vi "inspector_state_queue_manager.vi"(8 "error in":errorcluster, 10 "State array in":cluster{"State Enum":T1, "variant":variant}[](array[cluster]), 11 "Inspector_state_queue in":refnum<queue>) -> (0 "error out":errorcluster, 3 "Inspector_state_queue out":refnum<queue>)   [LabVIEW 2010]
uses:
  typedefs/inspector_state_enum.ctl
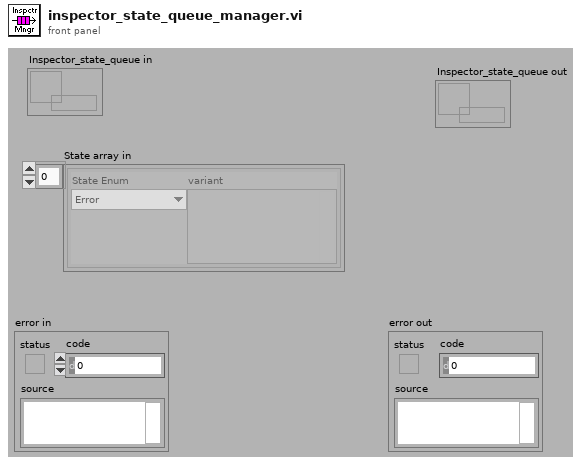
[diagram p1: front panel]
types:
  T1 = typedef "inspector_state_enum.ctl" = enum16{"Init", "Quit", "Error", "ZoomIn", "ZoomOut", "Load", "Change_channel", "Update_graphs"}
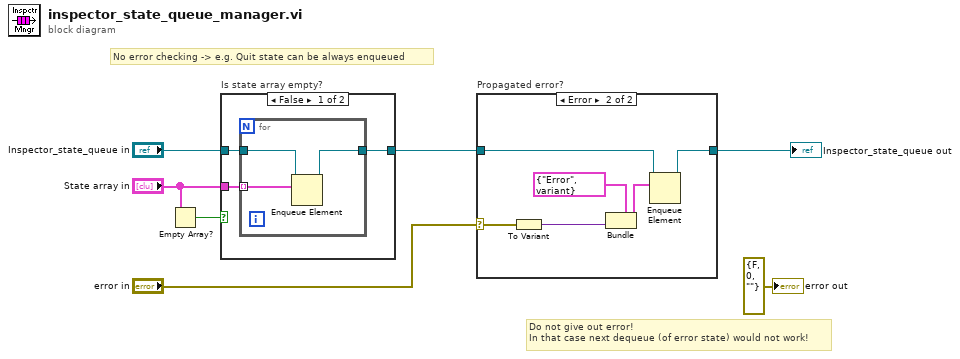
[diagram p0: block diagram]
diagram:
  # "Do not give out error!\nIn that case next dequeue (of error state) would not work!"
  # "No error checking -> e.g. Quit state can be always enqueued"
  n1 = Empty Array?(array="State array in") -> (empty?=w7:bool)
  n2 = case "Is state array empty?" shown="False" w7 {
    tunnel: "Inspector_state_queue in" -> [w10 w14]
    tunnel: [w9 w14] -> w5
    tunnel: "State array in" -> [w8 _]
    frame False {
      n3 = for {
        tunnel: w10 -> [w13]
        tunnel: w8 -> [w12] mode=indexing
        tunnel: [w11] -> w9
        n4 = Enqueue Element(queue=w13, element=w12) -> (queue out=w11:refnum<queue>)  [unwired: 2 in, 2 out]
      }
    }
    frame True {
      # "Empty state array?\nDo not call enqueue\nto avoid errors"
    }
  }
  n5 = case "Propagated error?" shown="Error" "error in" {
    selector: "error in" -> [_ w19]
    tunnel: w5 -> [w15 w21]
    tunnel: [w15 w20] -> w2
    frame No Error {
    }
    frame Error {
      n6 = To Variant(anything=w19) -> (Variant=w17:variant)
      n7 = Bundle(cluster=cluster{"State Enum":T1, "variant":variant} {"State Enum"=enum."Error", "variant"=variant} ("element"), "variant"=w17) -> (w16:cluster{"State Enum":T1, "variant":variant})  [unwired: 1 in]
      n8 = Enqueue Element(queue=w21, element=w16) -> (queue out=w20:refnum<queue>)  [unwired: 2 in, 2 out]
    }
  }
  "Inspector_state_queue out" <- w2
  "error out" <- errorcluster {"status"=FALSE, "code"=0, "source"=""} ("error out")
